vi "Actor Core.vi"(8 "error in":errorcluster, 11 "Nested in":refnum<class "Communicator Worker.lvclass">) -> (0 "error out":errorcluster, 3 "Actor out":refnum<class "Actor.lvclass">)   [LabVIEW 2019, in "Communicator Worker.lvlib" / "Communicator Worker.lvclass"]
doc: "(<B>Filename</B>: Actor Framework.lvlib:Actor.lvclass:Actor Core.vi)\n\nReceives messages to the actor, reacts to them, and initiates any error handling that may shut the actor down.\n\nDescendant classes may override this VI to append parallel tasks for the actor to complete while it handles messages. Overrides use the Call Parent Method node."
uses:
  Communicator Worker.lvclass
  Communicator Worker.lvclass/Communicator Worker.ctl
  Communicator Worker Messages/Read Messages Msg/Read Messages Msg.lvclass
  <vilib>/ActorFramework/Actor/Actor.lvclass
  <vilib>/ActorFramework/Actor Framework.lvlib
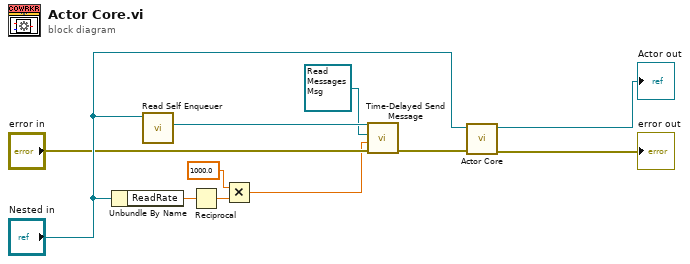
[diagram p0: block diagram]
diagram:
  n1 = Unbundle By Name("Nested in") -> ("ReadRate"=w9:dbl)
  n2 = call <vilib>:"Read Self Enqueuer.vi"("Actor"="Nested in") -> ("Self Enqueuer"=w5:refnum<class "Message Enqueuer.lvclass">)  [unwired: 10 in]
  n3 = Reciprocal(x=w9) -> (1/x=w8:dbl)
  n4 = Multiply(x=1000.0, y=w8) -> (x*y=w2:dbl)
  n5 = call <vilib>:"Time-Delayed Send Message.vi"("error in (no error)"="error in", "Milliseconds To Wait"=w2, "Message"=refnum<class "Read Messages Msg.lvclass"> refnum ("Communicator Worker.lvlib:Read Messages Msg.lvclass"), "Message Enqueuer"=w5) -> ("error out"=w3:errorcluster)  [unwired: 6 in, 1 out]
  n6 = call-parent "Actor Core.vi"("error in"=w3, "Actor in"="Nested in") -> ("error out"=→"error out":errorcluster, "Actor out"=→"Actor out":refnum<class "Actor.lvclass">)  [unwired: 8 in]
